vi "ScanParam2DAQParam.vi"(8 "error in":errorcluster, 11 "AOL_Globals":T1={"Imaging Protocol"=enum."AOL Z-Stack", "Number of POI"=0, "Number of Miniscans"=0, "Number of Trials"=0, "Number of Cycles "=0, "# Averaged Frames"=0, "Laser power (%)"=0, "Pockels (V)"=0.0, "Acquisition Length (sec)"=0.0, "Fill time (us)"=0.0, "POI Dwell time (us)"=0.0, "Miniscan Dwell time per pixel (us)"=0.0, "PMT 1"=0.0, "PMT 2"=0.0, "Back Apperture (mA)"=200.0, "Frame Size"=0, "Center Frequency"=0.0, "Field of View (um)"=175.0, "Field of View (norm)"=0.0, "DwellTime (us)"=0.0, "Ref Dwell Time (us)"=0.0, "Wavelength (nm)"=0.0, "Zoom"=0.0, "AOL Z"=0.0, "AOL Mode"=enum."Raster", "GridXY"=0.0, "GridZ"=0.0, "TriggerPeriod (sec)"=0.0, "Number of Pixels in Miniscan"=0, "Experiment folder path"=path "", "X centre"=0.0, "Y centre"=0.0, "Angle (degrees)"=0.0, "Angle Xs (degrees)"=0.0, "Angle Ys (degrees)"=0.0, "Plane Mode"=0, "Threshold"=[], "Regenerate Chirps"=FALSE, "Rectangle ROI length (pixels)"=0, "Rectangle ROI height (pixels)"=0, "AOD fill"=4900, "StartupDelay"=0, "Samples Wait after Trigger"=5080, "Slip Cycle"=600000, "Add Cycle"=TRUE, "Functional Mode"=enum."Point", "Z Start"=0.0, "Z Stop"=0.0, "# Planes"=0, "Total Pixels"=0, "Variable Miniscan Pixels"=[], "Use Variable Length"=FALSE, "Use Variable Resolution"=FALSE, "Laser power (%) at Z Start"=0, "Laser power (%) at Z Stop"=0, "Ref Z Step"=0} {"Angle Ys (degrees)" format="%#.6g"; "Angle Xs (degrees)" format="%#.6g"; "Plane Mode" items=["XY Plane", "XZ Plane", "YZ Plane", "arbitraryplane"]; "Frame Size" items=["100X100"=100, "128X128"=128, "200X200"=200, "256X256"=256, "512X512"=512, "1024x1024"=1024, "2048x2048"=2048]; "Back Apperture (mA)" format="%#.6g"; "Pockels (V)" format="%#.6g"; "PMT 2" format="%#.6g"; "PMT 1" format="%#.6g"; "Angle (degrees)" format="%#.6g"; "POI Dwell time (us)" format="%#.6g"}) -> (0 "error out":errorcluster, 3 "DAQ Input Parameters(FlexRIO)":T7 {"diff_threshZ" format="%#_11g"; "proportioanl_scale Z" format="%#_15g"; "var_x" format="%#_14g"; "var_y" format="%#_14g"; "scale" format="%#_15g"; "diff_thresh" format="%#_11g"; "proportioanl_scale" format="%#_15g"})   [LabVIEW 2020]
uses:
  Typedefs/Controls/DAQ Input Parameters(FlexRIO).ctl
  FPGA Host VIs/typedefs/scan_type.ctl
  Movement Correction/Typedefs/Control algorithm.ctl
  Typedefs/Controls/AOL_Globals.ctl
  Typedefs/Imaging Protocols enum.ctl
  Typedefs/Frame Size.ctl
  Typedefs/AOL modes.ctl
  Typedefs/Plane Mode.ctl
  Typedefs/Functional Mode.ctl
  Global Variables/General Globals.vi
panel:
  out "Number of Cycles":u64
  out "Repeat (Number of Cycles)":u32
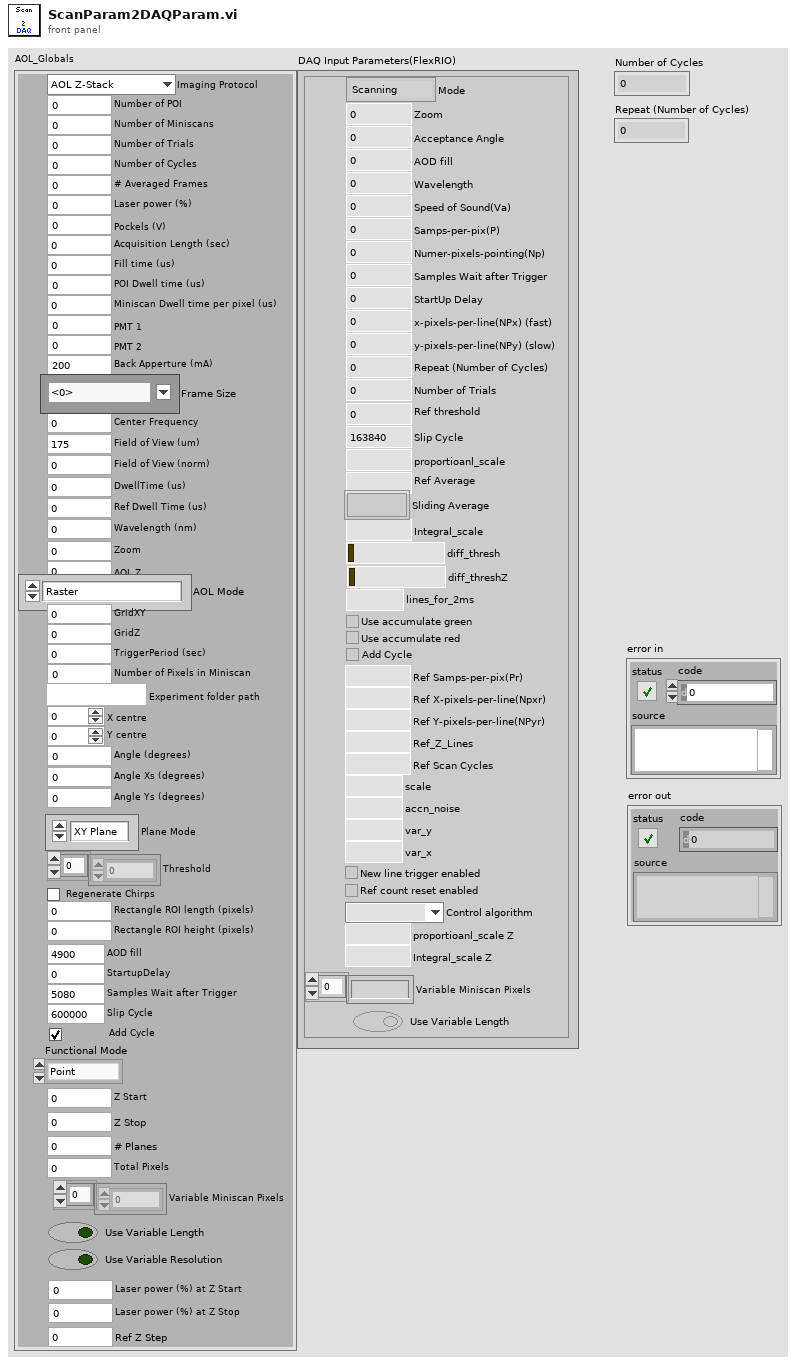
[diagram p1: front panel]
types:
  T1 = typedef "AOL_Globals.ctl" = cluster{"Imaging Protocol":T2, "Number of POI":u16, "Number of Miniscans":u16, "Number of Trials":u16, "Number of Cycles ":u64, "# Averaged Frames":u16, "Laser power (%)":u8, "Pockels (V)":dbl, "Acquisition Length (sec)":dbl, "Fill time (us)":dbl, "POI Dwell time (us)":dbl, "Miniscan Dwell time per pixel (us)":dbl, "PMT 1":dbl, "PMT 2":dbl, "Back Apperture (mA)":dbl, "Frame Size":T3, "Center Frequency":dbl, "Field of View (um)":dbl, "Field of View (norm)":dbl, "DwellTime (us)":dbl, "Ref Dwell Time (us)":dbl, "Wavelength (nm)":dbl, "Zoom":dbl, "AOL Z":dbl, "AOL Mode":T4, "GridXY":dbl, "GridZ":dbl, "TriggerPeriod (sec)":dbl, "Number of Pixels in Miniscan":u16, "Experiment folder path":path, "X centre":dbl, "Y centre":dbl, "Angle (degrees)":dbl, "Angle Xs (degrees)":dbl, "Angle Ys (degrees)":dbl, "Plane Mode":T5, "Threshold":u16[], "Regenerate Chirps":bool, "Rectangle ROI length (pixels)":u16, "Rectangle ROI height (pixels)":u16, "AOD fill":u16, "StartupDelay":i32, "Samples Wait after Trigger":u16, "Slip Cycle":u32, "Add Cycle":bool, "Functional Mode":T6, "Z Start":dbl, "Z Stop":dbl, "# Planes":i32, "Total Pixels":i32, "Variable Miniscan Pixels":u16[], "Use Variable Length":bool, "Use Variable Resolution":bool, "Laser power (%) at Z Start":u8, "Laser power (%) at Z Stop":u8, "Ref Z Step":i8}
  T2 = typedef "Imaging Protocols enum.ctl" = enum16{"AOL Z-Stack", "Motor Z Stack", "Parameter Sweep", "Functional Acquisition", "Single Plane Acquisition", "Volume Acquisition", "Live Imaging", "Live Plane Imaging", "Live Volume Imaging"}
  T3 = typedef "Frame Size.ctl" = u16
  T4 = typedef "AOL modes.ctl" = enum16{"Raster", "Structural", "Pointing", "Mini Scan", "Alignment"}
  T5 = typedef "Plane Mode.ctl" = u16
  T6 = typedef "Functional Mode.ctl" = enum16{"Point", "Line", "Patch", "Plane", "Volume"}
  T7 = typedef "DAQ Input Parameters(FlexRIO).ctl" = cluster{"Mode":T8, "Zoom":i8, "Acceptance Angle":i8, "AOD fill":u16, "Wavelength":i16, "Speed of Sound(Va)":i8, "Samps-per-pix(P)":i16, "Numer-pixels-pointing(Np)":u32, "Samples Wait after Trigger":u16, "StartUp Delay":i32, "x-pixels-per-line(NPx) (fast)":u16, "y-pixels-per-line(NPy) (slow)":u16, "Repeat (Number of Cycles)":u32, "Number of Trials":u16, "Ref threshold":u16, "Slip Cycle":u32, "proportioanl_scale":fxp<+,16,2>, "Ref Average":u16, "Sliding Average":bool, "Integral_scale":fxp<+/-,16,12>, "diff_thresh":fxp<+/-,16,8>, "diff_threshZ":fxp<+/-,16,8>, "lines_for_2ms":i16, "Use accumulate green":bool, "Use accumulate red":bool, "Add Cycle":bool, "Ref Samps-per-pix(Pr)":i16, "Ref X-pixels-per-line(Npxr)":i16, "Ref Y-pixels-per-line(NPyr)":i16, "Ref_Z_Lines":i16, "Ref Scan Cycles":i32, "scale":fxp<+,16,2>, "accn_noise":fxp<+,16,16>, "var_y":fxp<+,16,4>, "var_x":fxp<+,16,4>, "New line trigger enabled":bool, "Ref count reset enabled":bool, "Control algorithm":T9, "proportioanl_scale Z":fxp<+,16,2>, "Integral_scale Z":fxp<+/-,16,12>, "Variable Miniscan Pixels":u16[], "Use Variable Length":bool}
  T8 = typedef "scan_type.ctl" = enum16{"Scanning", "Pointing", "Pointing & MC", "Scanning & MC"}
  T9 = typedef "Control algorithm.ctl" = enum16{"PID", "Kalman"}
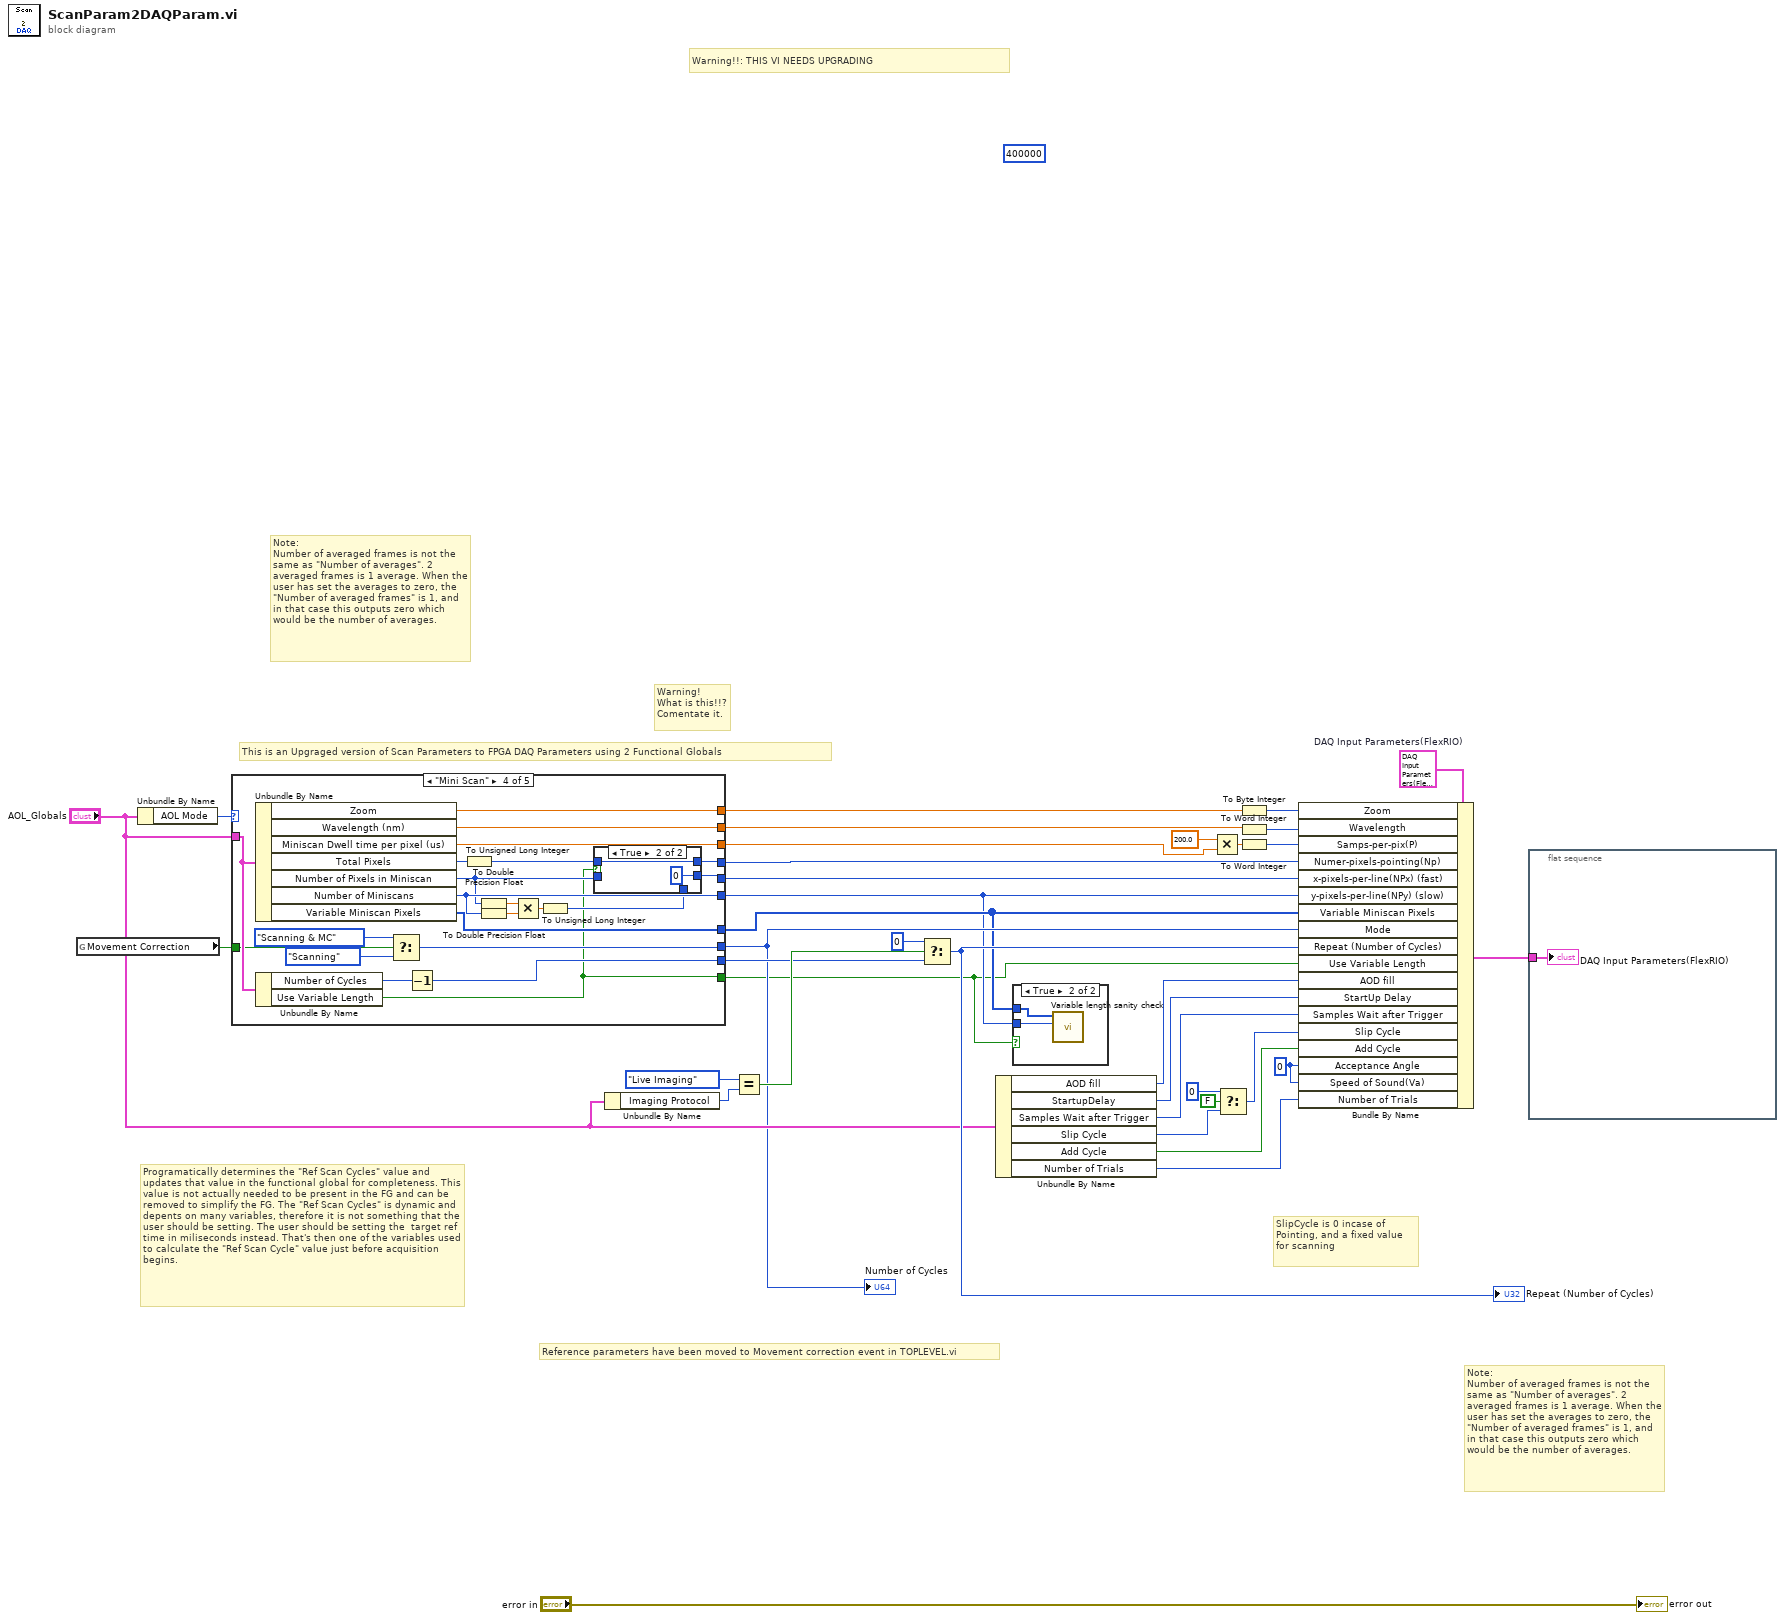
[diagram p0: block diagram]
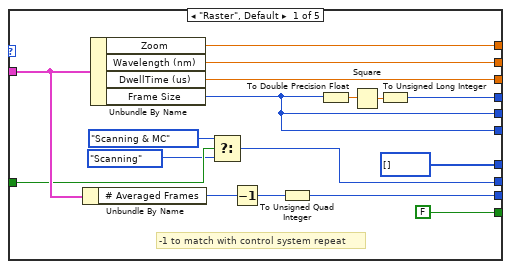
[diagram p3: hidden frame]
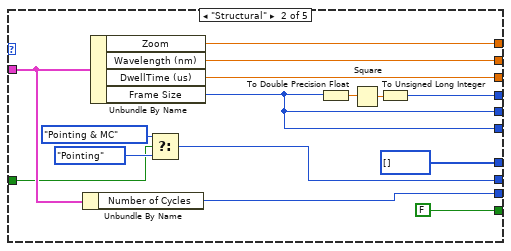
[diagram p4: hidden frame]
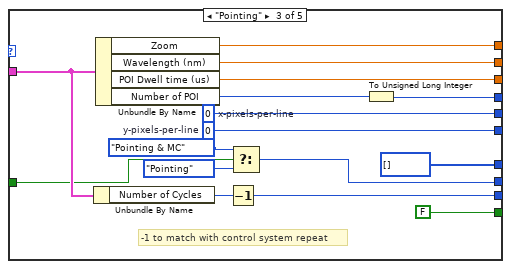
[diagram p5: hidden frame]
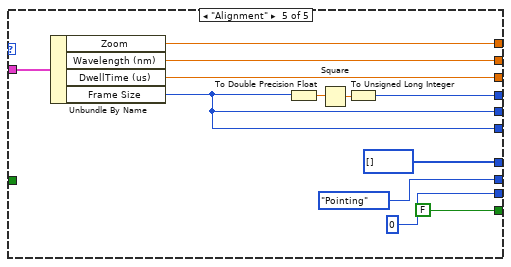
[diagram p7: hidden frame]
diagram:
  w10 = i8 0 ("Speed of Sound(Va)")
  w14 = T7 data[162B]  # DAQ Input Parameters(FlexRIO)
  (unwired) 400000 ("Ref Scan Cycles")
  # "Reference parameters have been moved to Movement correction event in TOPLEVEL.vi"
  # "Programatically determines the \"Ref Scan Cycles\" value and updates that value in the functional global for completeness. This value is not actually needed to be present in the FG and can be removed to simplify the FG. The \"Ref Scan Cycles\" is dynamic and depents on many variables, therefore it is not something that the user should be setting. The user should be setting the  target ref time in miliseconds instead. That's then one of the variables used to calculate the \"Ref Scan Cycle\" value just before acquisition begins."
  # "Warning!\nWhat is this!!?\nComentate it."
  # "Note:\nNumber of averaged frames is not the same as \"Number of averages\". 2 averaged frames is 1 average. When the user has set the averages to zero, the \"Number of averaged frames\" is 1, and in that case this outputs zero which would be the number of averages."
  # "SlipCycle is 0 incase of Pointing, and a fixed value for scanning"
  # "Note:\nNumber of averaged frames is not the same as \"Number of averages\". 2 averaged frames is 1 average. When the user has set the averages to zero, the \"Number of averaged frames\" is 1, and in that case this outputs zero which would be the number of averages."
  # "This is an Upgraged version of Scan Parameters to FPGA DAQ Parameters using 2 Functional Globals"
  # "Warning!!: THIS VI NEEDS UPGRADING"
  n1 = global read "General Globals.vi" "Movement Correction"() -> (w24:bool)
  n2 = Unbundle By Name("AOL_Globals") -> ("AOL Mode"=w36:T4)
  n3 = case shown="\"Mini Scan\"" w36 {
    tunnel: "AOL_Globals" -> [w47 w61 w78 w103 w122]
    tunnel: [w53 w68 w84 w106 w121] -> w35
    tunnel: [w52 w67 w83 w105 w120] -> w30
    tunnel: [w49 w64 w82 w104 w117] -> w27
    tunnel: [w48 w63 w80 w88 w116] -> w28
    tunnel: [w48 w63 w79 w100 w116] -> w2
    tunnel: [w44 w60 w75 w94 scan_type."Pointing" ("Mode")] -> w4
    tunnel: [w40 w57 w76 w99 u64 0 ("Number of Cycles")] -> w5
    tunnel: w24 -> [w46 w58 w73 w96 _]
    tunnel: [w39 w56 w71 w89 w113] -> w6
    tunnel: [u16[] [] ("Variable Miniscan Pixels") u16[] [] ("Variable Miniscan Pixels") u16[] [] ("Variable Miniscan Pixels") w91 u16[] [] ("Variable Miniscan Pixels")] -> w3
    tunnel: [FALSE ("Use Variable Length") FALSE ("Use Variable Length") FALSE ("Use Variable Length") w85 FALSE ("Use Variable Length")] -> w1
    frame "Raster", Default {
      # "-1 to match with control system repeat"
      n4 = Unbundle By Name(w47) -> ("# Averaged Frames"=w42:u16)
      n5 = Unbundle By Name(w47) -> ("Zoom"=w53:dbl, "Wavelength (nm)"=w49:dbl, "DwellTime (us)"=w52:dbl, "Frame Size"=w48:T3)
      n6 = Select(t=scan_type."Scanning & MC" ("Mode"), s=w46, f=scan_type."Scanning" ("Mode")) -> (s? t:f=w44:T8)
      n7 = Decrement(x=w42) -> (x-1=w41:u16)
      n8 = To Unsigned Quad Integer(1:w41) -> (0:w40:u64)
      n9 = To Double Precision Float(number=w48) -> (double precision float=w51:dbl)
      n10 = Square(x=w51) -> (x^2=w50:dbl)
      n11 = To Unsigned Long Integer(number=w50) -> (unsigned 32bit integer=w39:u32)
    }
    frame "Structural" {
      n12 = Unbundle By Name(w61) -> ("Number of Cycles"=w57:u64)
      n13 = Unbundle By Name(w61) -> ("Zoom"=w68:dbl, "Wavelength (nm)"=w64:dbl, "DwellTime (us)"=w67:dbl, "Frame Size"=w63:T3)
      n14 = Select(t=scan_type."Pointing & MC" ("Mode"), s=w58, f=scan_type."Pointing" ("Mode")) -> (s? t:f=w60:T8)
      n15 = To Double Precision Float(number=w63) -> (double precision float=w66:dbl)
      n16 = Square(x=w66) -> (x^2=w65:dbl)
      n17 = To Unsigned Long Integer(number=w65) -> (unsigned 32bit integer=w56:u32)
    }
    frame "Pointing" {
      w79 = u16 0  # y-pixels-per-line
      w80 = u16 0  # x-pixels-per-line
      # "-1 to match with control system repeat"
      n18 = Unbundle By Name(w78) -> ("Number of Cycles"=w77:u64)
      n19 = Unbundle By Name(w78) -> ("Zoom"=w84:dbl, "Wavelength (nm)"=w82:dbl, "POI Dwell time (us)"=w83:dbl, "Number of POI"=w72:u16)
      n20 = Decrement(x=w77) -> (x-1=w76:u64)
      n21 = Select(t=scan_type."Pointing & MC" ("Mode"), s=w73, f=scan_type."Pointing" ("Mode")) -> (s? t:f=w75:T8)
      n22 = To Unsigned Long Integer(number=w72) -> (unsigned 32bit integer=w71:u32)
    }
    frame "Mini Scan" {
      n23 = Unbundle By Name(w103) -> ("Zoom"=w106:dbl, "Wavelength (nm)"=w104:dbl, "Miniscan Dwell time per pixel (us)"=w105:dbl, "Total Pixels"=w92:i32, "Number of Pixels in Miniscan"=w86:u16, "Number of Miniscans"=w100:u16, "Variable Miniscan Pixels"=w91:u16[])
      n24 = Unbundle By Name(w103) -> ("Number of Cycles"=w102:u64, "Use Variable Length"=w85:bool)
      n25 = Select(t=scan_type."Scanning & MC" ("Mode"), s=w96, f=scan_type."Scanning" ("Mode")) -> (s? t:f=w94:T8)
      n26 = Decrement(x=w102) -> (x-1=w99:u64)
      n27 = To Unsigned Long Integer(number=w92) -> (unsigned 32bit integer=w90:u32)
      n28 = To Double Precision Float(number=w86) -> (double precision float=w98:dbl)
      n29 = To Double Precision Float(number=w100) -> (double precision float=w97:dbl)
      n30 = Multiply(x=w98, y=w97) -> (x*y=w101:dbl)
      n31 = To Unsigned Long Integer(number=w101) -> (unsigned 32bit integer=w87:u32)
      n32 = case shown="True" w85 {
        tunnel: w90 -> [_ w110]
        tunnel: [w108 w110] -> w89
        tunnel: [w107 0] -> w88
        tunnel: w87 -> [w108 _]
        tunnel: w86 -> [w107 _]
        frame False {
        }
        frame True {
        }
      }
    }
    frame "Alignment" {
      n33 = Unbundle By Name(w122) -> ("Zoom"=w121:dbl, "Wavelength (nm)"=w117:dbl, "DwellTime (us)"=w120:dbl, "Frame Size"=w116:T3)
      n34 = To Double Precision Float(number=w116) -> (double precision float=w119:dbl)
      n35 = Square(x=w119) -> (x^2=w118:dbl)
      n36 = To Unsigned Long Integer(number=w118) -> (unsigned 32bit integer=w113:u32)
    }
  }
  "Number of Cycles" <- w4
  n37 = Unbundle By Name("AOL_Globals") -> ("Imaging Protocol"=w21:T2)
  n38 = Equal?(x=Imaging_Protocols_enum."Live Imaging", y=w21) -> (x = y?=w22:bool)
  n39 = Select(t=u64 0, s=w22, f=w5) -> (s? t:f=w18:u64)
  "Repeat (Number of Cycles)" <- w18
  n40 = Unbundle By Name("AOL_Globals") -> ("AOD fill"=w13:u16, "StartupDelay"=w17:i32, "Samples Wait after Trigger"=w8:u16, "Slip Cycle"=w12:u32, "Add Cycle"=w16:bool, "Number of Trials"=w7:u16)
  n41 = case shown="True" w1 {
    tunnel: w3 -> [_ w124]
    tunnel: w2 -> [_ w123]
    frame False {
    }
    frame True {
      n42 = call "Variable length sanity check.vi"("Number of miniscans"=w123, "VL X pixels"=w124) -> ()  [unwired: 10 in]
    }
  }
  n43 = Multiply(x=200.0, y=w30) -> (x*y=w33:dbl)
  n44 = Select(t=u32 0, s=FALSE, f=w12) -> (s? t:f=w11:u32)
  n45 = To Byte Integer(number=w35) -> (8bit integer=w34:i8)
  n46 = To Word Integer(number=w27) -> (16bit integer=w29:i16)
  n47 = To Word Integer(number=w33) -> (16bit integer=w31:i16)
  n48 = Bundle By Name(cluster=w14, "Zoom"=w34, "Wavelength"=w29, "Samps-per-pix(P)"=w31, "Numer-pixels-pointing(Np)"=w6, "x-pixels-per-line(NPx) (fast)"=w28, "y-pixels-per-line(NPy) (slow)"=w2, "Variable Miniscan Pixels"=w3, "Mode"=w4, "Repeat (Number of Cycles)"=w18, "Use Variable Length"=w1, "AOD fill"=w13, "StartUp Delay"=w17, "Samples Wait after Trigger"=w8, "Slip Cycle"=w11, "Add Cycle"=w16, "Acceptance Angle"=w10, "Speed of Sound(Va)"=w10, "Number of Trials"=w7) -> (w9:T7)
  n49 = flat-sequence {
    tunnel: w9 -> [w125]
    frame #0 {
      "DAQ Input Parameters(FlexRIO)" <- w125
    }
  }
  "error out" <- "error in"
